vi "Prevent Overscroll.vi"(8 "error in (no error)":errorcluster, 11 "Array Refnum":refnum<vi>) -> (0 "error out":errorcluster, 3 "Array Refnum":refnum<vi>)   [LabVIEW 2017, in "UI Common.lvlib"]
uses:
  UI Common.lvlib
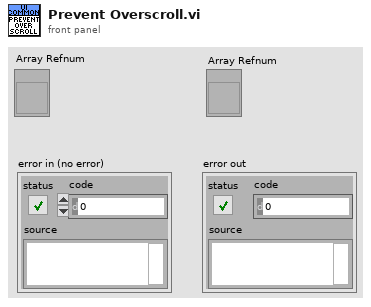
[diagram p1: front panel]
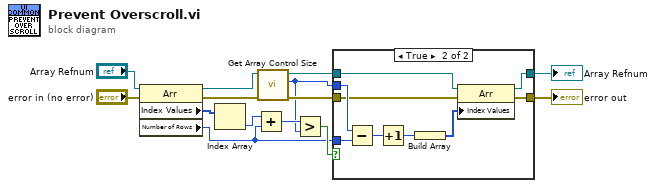
[diagram p0: block diagram]
diagram:
  n1 = property class="Arr"(reference="Array Refnum", error in="error in (no error)") -> (reference out=w5:refnum<vi>, error out=w6:errorcluster, "Index Values"=w4:u32[], "Number of Rows"=w2:u32)
  n2 = Index Array(array=w4) -> (element=w3:u32)  [unwired: 1 in]
  n3 = Add(x=w3, y=w2) -> (x+y=w10:u32)
  n4 = call "Get Array Control Size.vi"("error in (no error)"=w6, "Array in"=w5) -> ("error out"=w9:errorcluster, "Size"=w1:i32, "Array out"=w13:refnum<vi>)  [unwired: 7 in]
  n5 = Greater?(x=w10, y=w1) -> (0:w12:bool)
  n6 = case shown="True" w12 {
    tunnel: w13 -> [w15 w19]
    tunnel: w9 -> [w16 w21]
    tunnel: [w16 w20] -> w14
    tunnel: [w15 w17] -> w11
    tunnel: w2 -> [_ w25]
    tunnel: w1 -> [_ w24]
    frame False {
    }
    frame True {
      n7 = Subtract(x=w24, y=w25) -> (x-y=w23:u32)
      n8 = Increment(x=w23) -> (x+1=w22:u32)
      n9 = Build Array(w22) -> (w18:u32[])
      n10 = property class="Arr"(reference=w19, error in=w21, "Index Values"=w18) -> (reference out=w17:refnum<vi>, error out=w20:errorcluster)
    }
  }
  "error out" <- w14
  "Array Refnum" <- w11
